vi "运维调试_质控单元.vi"() -> ()   [LabVIEW 2016, in "质控单元.lvlib"]
uses:
  <vilib>/Utility/miscctls.llb/LVPointTypeDef.ctl
  <vilib>/Plasmionique/MB Master/MB_Master_Serial/MB_Master_Serial.lvclass
  C:/Program Files (x86)/National Instruments/LabVIEW 2016/vi.lib/Plasmionique/MB Master/MB_Master/MB_Master.lvclass
  <vilib>/Plasmionique/MB Master/MB Master.lvlib
  <vilib>/ptbypt/NI_PtbyPt.lvlib
panel:
  out "启动模块":T1
  out "COD传感器故障报警":bool
  in  "总氮停止":bool
  in  "总氮排液":bool
  in  "总氮调试":bool
  out "总氮加标回收率":dbl caption="加标回收率" format="%.2f"
  out "总氮加标体积":dbl caption="加标体积" format="%.3f"
  out "总氮母液浓度":dbl caption="加标母液浓度" format="%.3f"
  out "总氮加标水杯定容体积":dbl caption="加标水杯定容体积" format="%.2f"
  out "总氮加标后水样浓度":dbl caption="加标后水样浓度" format="%.3f"
  out "总氮加标前水样浓度":dbl caption="加标前水样浓度" format="%.3f"
  out "总氮检出限":dbl caption="检出限" format="%.3f"
  out "总氮量程":dbl caption="量程" format="%.2f"
  out "总氮状态":u16(ring) caption="状态" items=["待机", "润洗", "进样", "等待取液", "排液"]
  in  "返回":bool
  in  "查看":bool
  out "COD液位传感器":bool
  out "氨氮总磷液位传感器":bool
  out "直接启动":bool
  out "常规启动":bool
  out "总磷总氮传感器故障报警":bool
  out "氨氮传感器故障报警":bool
  out "columns":string[](array[string])
  out "data":T2
  out "氨氮加标回收测完标志":bool
  out "COD加标回收测完标志":bool
  out "氨氮总磷加标回收测完标志":bool
  out "COD平行样测完标志":bool
  out "氨氮总磷平行样测完标志":bool
  out "输出簇 2":T3
  out "常规启动 2":bool
  out "直接启动 2":bool
  out "启动模块 2":cluster{"氨氮1":bool, "总磷1":bool, " COD1":bool}
  in  "停止测量":bool
  out "输出簇":T4
  in  "启动流程":T5(ring)
  in  "加标回收":bool
  in  "平行样测试":bool
  in  "CODMn停止":bool
  in  "CODMn排液":bool
  in  "CODMn调试":bool
  in  "总磷停止":bool
  in  "总磷排液":bool
  in  "总磷调试":bool
  out "COD加标回收率":dbl caption="加标回收率" format="%.2f"
  out "COD加标体积":dbl caption="加标体积" format="%.3f"
  out "COD母液浓度":dbl caption="加标母液浓度" format="%.2f"
  out "COD加标水杯定容体积":dbl caption="加标水杯定容体积" format="%.2f"
  out "COD加标后水样浓度":dbl caption="加标后水样浓度" format="%.2f"
  out "COD加标前水样浓度":dbl caption="加标前水样浓度" format="%.2f"
  out "COD检出限":dbl caption="检出限" format="%.2f"
  out "COD量程":dbl caption="量程" format="%.2f"
  out "COD状态":u16(ring) caption="状态" items=["待机", "润洗", "进样", "等待取液", "排液"]
  out "总磷加标回收率":dbl caption="加标回收率" format="%.2f"
  out "总磷加标体积":dbl caption="加标体积" format="%.3f"
  out "总磷母液浓度":dbl caption="加标母液浓度" format="%.3f"
  out "总磷加标水杯定容体积":dbl caption="加标水杯定容体积" format="%.2f"
  out "总磷加标后水样浓度":dbl caption="加标后水样浓度" format="%.3f"
  out "总磷加标前水样浓度":dbl caption="加标前水样浓度" format="%.3f"
  out "总磷检出限":dbl caption="检出限" format="%.3f"
  out "总磷量程":dbl caption="量程" format="%.2f"
  out "总磷状态":u16(ring) caption="状态" items=["待机", "润洗", "进样", "等待取液", "排液"]
  out "氨氮加标回收率":dbl caption="加标回收率" format="%.2f"
  out "氨氮加标体积":dbl caption="加标体积" format="%.3f"
  out "氨氮母液浓度":dbl caption="加标母液浓度" format="%.3f"
  out "氨氮加标水杯定容体积":dbl caption="加标水杯定容体积" format="%.2f"
  out "氨氮加标后水样浓度":dbl caption="加标后水样浓度" format="%.3f"
  out "氨氮加标前水样浓度":dbl caption="加标前水样浓度" format="%.3f"
  out "氨氮检出限":dbl caption="检出限" format="%.3f"
  out "氨氮量程":dbl caption="量程" format="%.2f"
  out "氨氮状态":u16(ring) caption="状态" items=["待机", "润洗", "进样", "等待取液", "排液"]
  in  "氨氮停止":bool
  in  "氨氮排液":bool
  in  "氨氮调试":bool
  # "总氮质控参数"
  # "%"
  # "mL"
  # "mg/L"
  # "mL"
  # "mg/L"
  # "mg/L"
  # "mg/L"
  # "mg/L"
  # "CODCr质控参数"
  # "%"
  # "mL"
  # "mg/L"
  # "mL"
  # "mg/L"
  # "mg/L"
  # "mg/L"
  # "mg/L"
  # "总磷质控参数"
  # "%"
  # "mL"
  # "mg/L"
  # "mL"
  # "mg/L"
  # "mg/L"
  # "mg/L"
  # "mg/L"
  # "氨氮质控参数"
  # "%"
  # "mL"
  # "mg/L"
  # "mL"
  # "mg/L"
  # "mg/L"
  # "mg/L"
  # "mg/L"
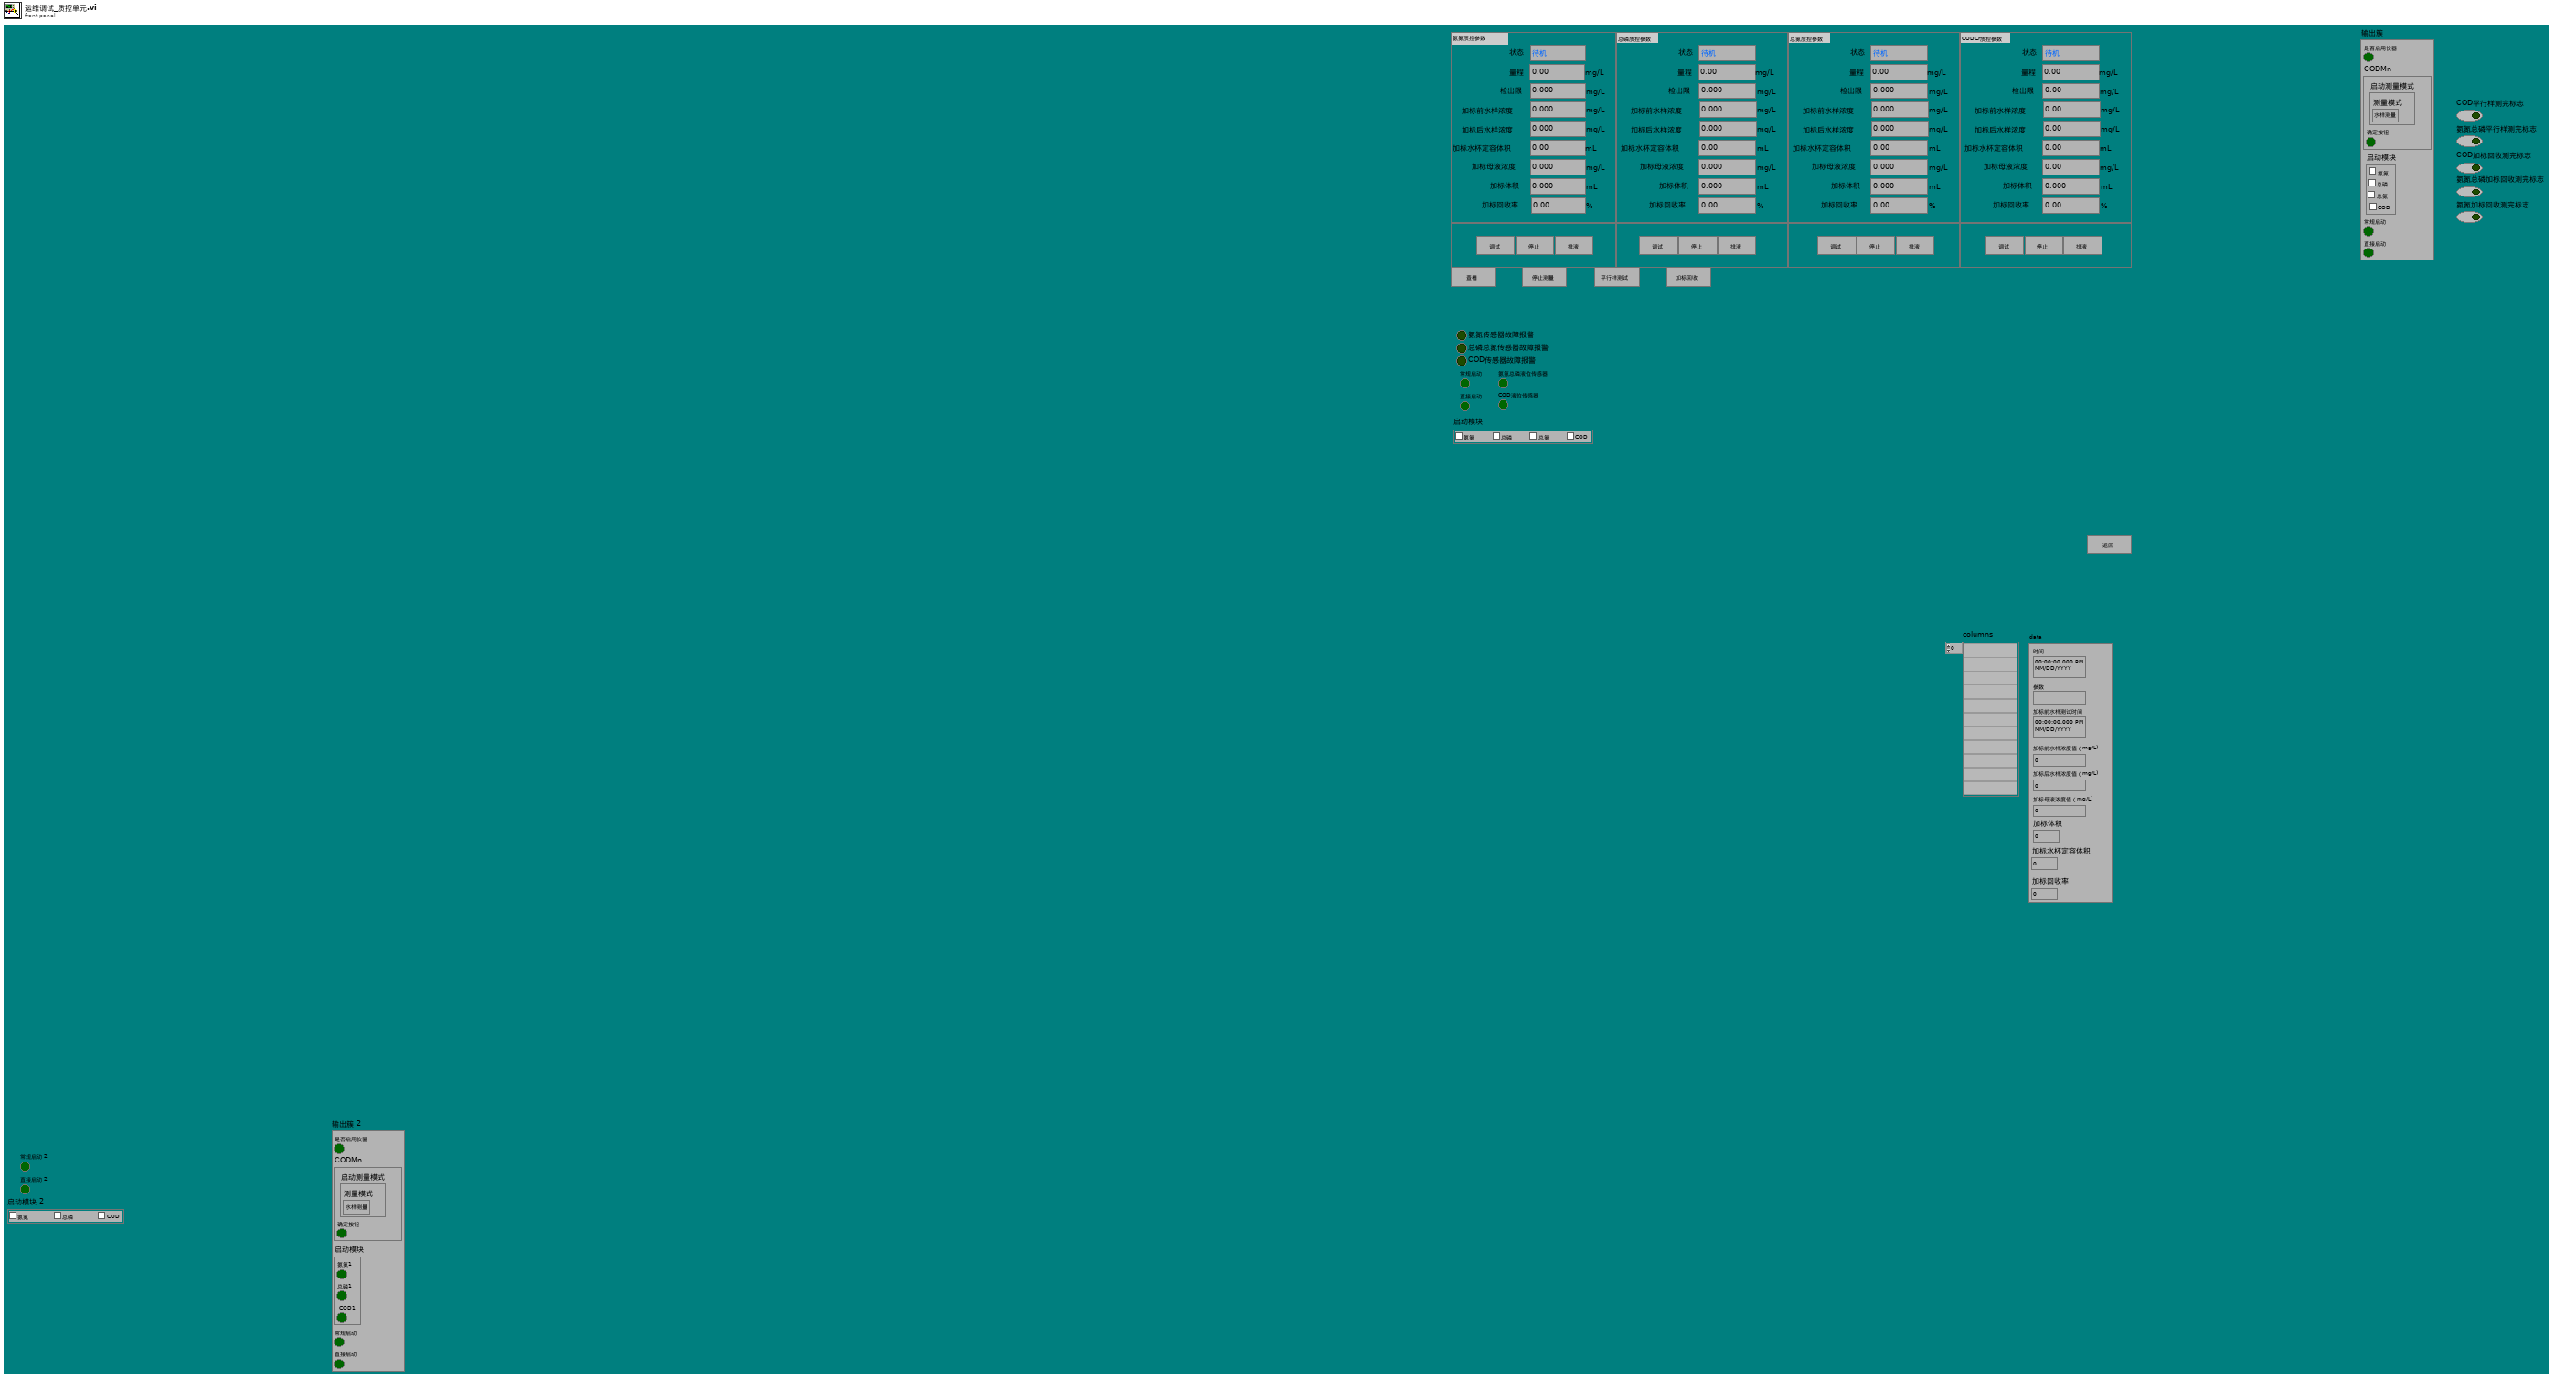
[diagram p1: front panel]
types:
  T1 = cluster{"氨氮":bool, "总磷":bool, "总氮":bool, "COD":bool}
  T2 = cluster{"时间":timestamp, "参数":string, "加标前水样测试时间":timestamp, "加标前水样浓度值（mg/L)":sgl, "加标后水样浓度值（mg/L)":sgl, "加标母液浓度值（mg/L)":sgl, "加标体积":dbl, "加标水杯定容体积":dbl, "加标回收率":dbl}
  T3 = cluster{"是否启用仪器":bool, "CODMn":cluster{"启动测量模式":cluster{"测量模式":enum16{"水样测量", "标样核查", "加标回收", "平行样", "校零", "校标"}}, "确定按钮":bool}, "启动模块":cluster{"氨氮1":bool, "总磷1":bool, " COD1":bool}, "常规启动":bool, "直接启动":bool}
  T4 = cluster{"是否启用仪器":bool, "CODMn":cluster{"启动测量模式":cluster{"测量模式":enum16{"水样测量", "标样核查", "加标回收", "平行样", "校零", "校标"}}, "确定按钮":bool}, "启动模块 3":cluster{"氨氮":bool, "总磷":bool, "总氮":bool, "COD":bool}, "常规启动":bool, "直接启动":bool}
  T5 = enum16{"初始化", "采配水", "测量水样", "加标", "取样测量", "测量结束"}
  T6 = typedef "LVPointTypeDef.ctl" = cluster{"Horizontal":i16, "Vertical":i16}
  T7 = cluster{"baud rate (bps)":u32, "stop bits":u16, "parity":u16, "flow control":u16, "timeout":u32, "retries":i32}
  T8 = cluster{"量程":dbl, "检出限":dbl, "加标前水样浓度":dbl, "加标后水样浓度":dbl, "加标水杯定容体积":dbl, "加标母液浓度":dbl, "加标体积":dbl, "加标回收率":dbl}
  T9 = cluster{"因子编码":u32, "单位":u16, "标样参考值":sgl, "水样数据时间":timestamp, "水样实测值":sgl, "水样数据标识":string, "标样数据时间":timestamp, "标样实测值":sgl, "标样数据标识":string, "空白数据时间":timestamp, "空白实测值":sgl, "空白数据标识":string, "零点核查数据时间":timestamp, "零点核查实测值":sgl, "零点核查数据标识":string, "跨度核查数据时间":timestamp, "跨度核查实测值":sgl, "跨度核查数据标识":string, "加标回收数据时间":timestamp, "加标回收实测值":sgl, "加标回收数据标识":string, "平行样数据时间":timestamp, "平行样实测值":sgl, "平行样数据标识":string, "F0":sgl, "F1":sgl, "F2":sgl, "F3":sgl, "F4":sgl, "F5":sgl, "F6":sgl, "F7":sgl, "温度":sgl, "湿度":sgl, "X值":sgl}
  T10 = cluster{"时间":timestamp, "测量模式":string, "数据类型":string, "检测值":sgl, "单位":string, "数据标识":string, "因子编码":string, "标样参考值":sgl, "ORP-A":sgl, "ORP-B":sgl, "ORP-K":sgl, "COD滴定值":sgl, "高锰酸钾滴定数":sgl, "温度":sgl}
  T11 = enum8{"Enabled", "Disabled", "Disabled and Grayed Out"}
  T12 = cluster{"命令":string, cluster{"starting address":u16, "holding register value":u16}}
  T13 = enum32{"Bad", "Idle", "Run top level", "Running"}
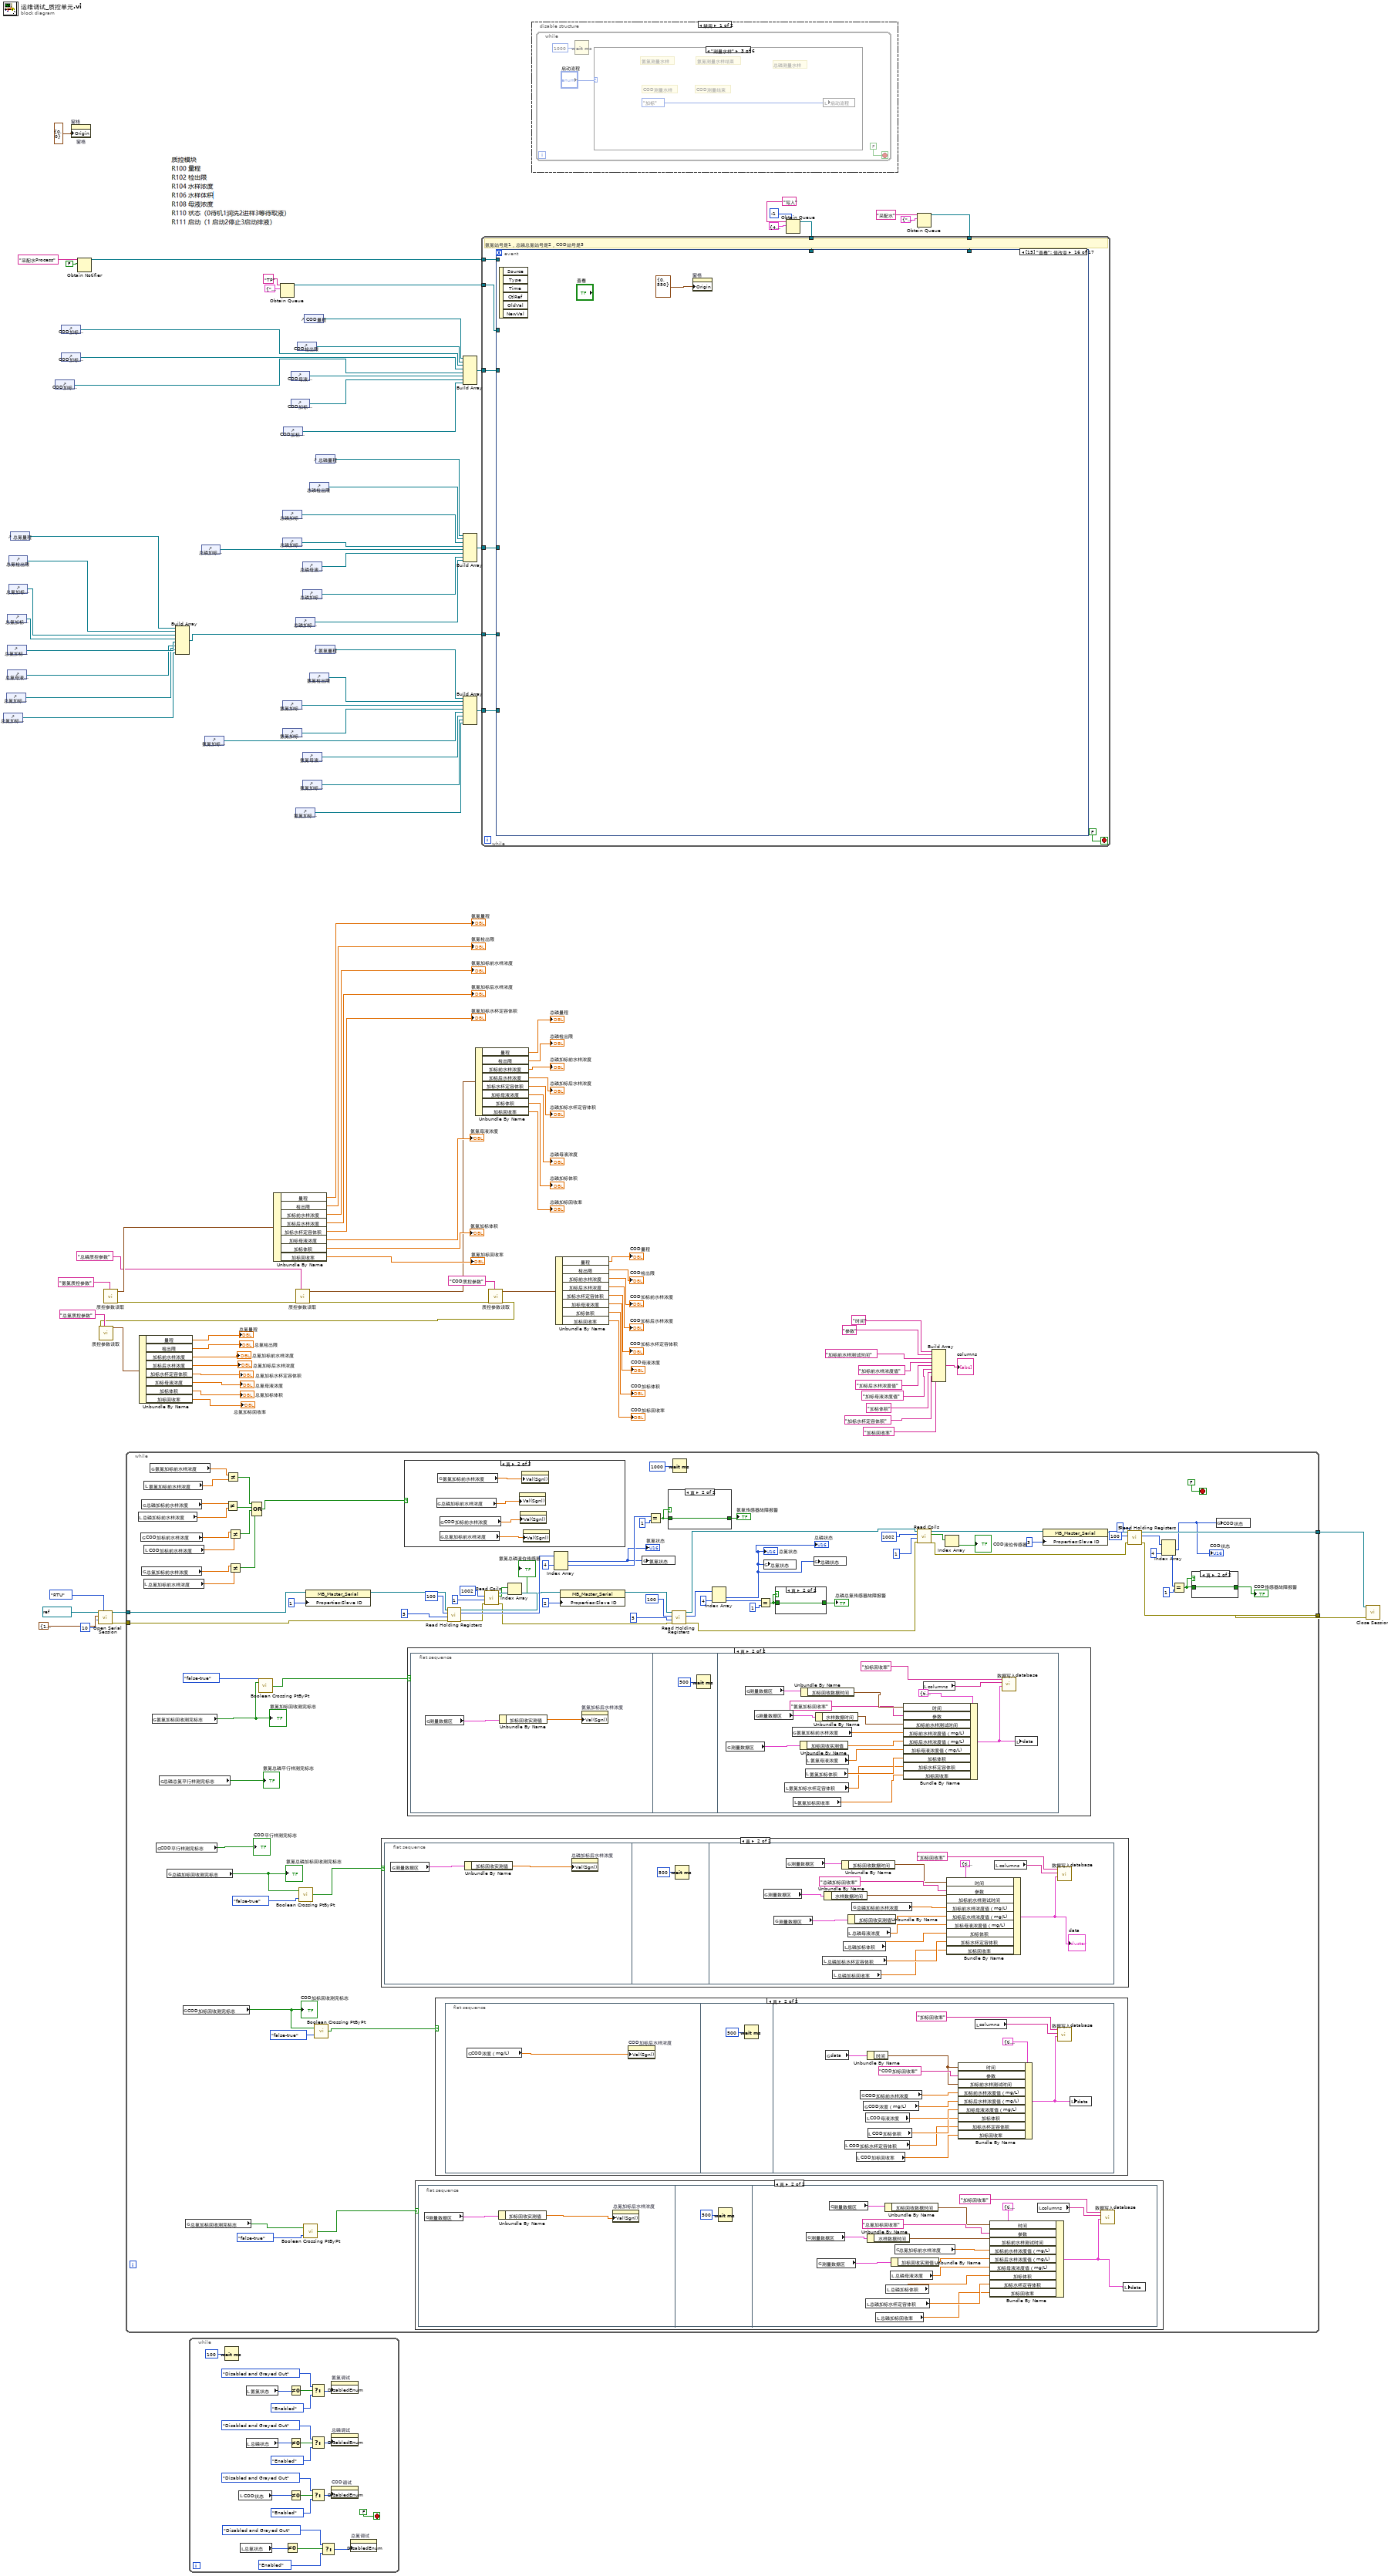
[diagram p0: block diagram]
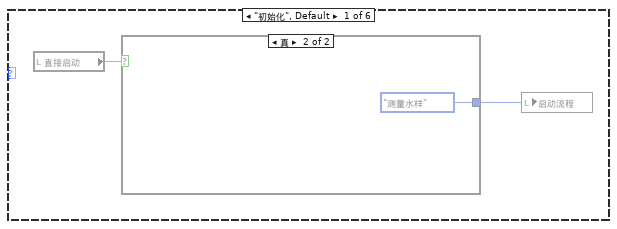
[diagram p2: hidden frame]
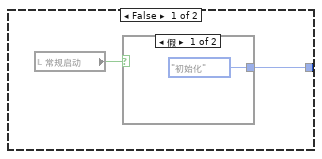
[diagram p3: hidden frame]
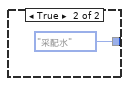
[diagram p4: hidden frame]
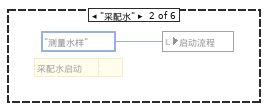
[diagram p5: hidden frame]
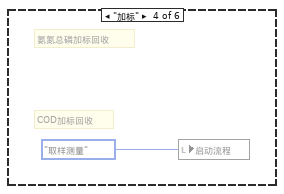
[diagram p6: hidden frame]
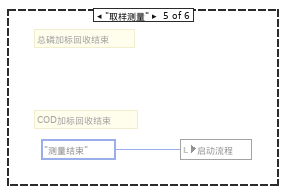
[diagram p7: hidden frame]
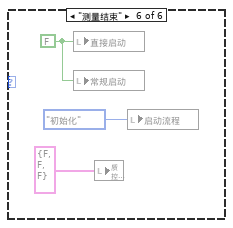
[diagram p8: hidden frame]
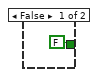
[diagram p11: hidden frame]
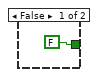
[diagram p16: hidden frame]
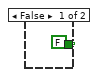
[diagram p17: hidden frame]
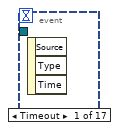
[diagram p18: hidden frame]
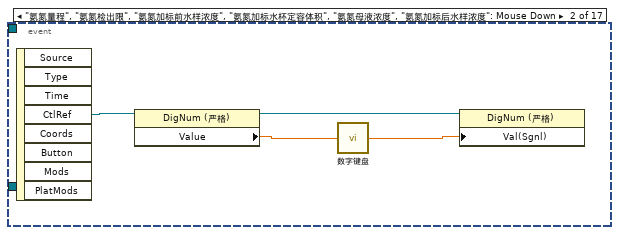
[diagram p19: hidden frame]
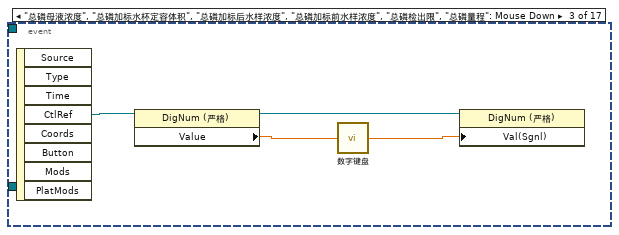
[diagram p20: hidden frame]
diagram:
  n1 = control-ref of="总氮加标回收率"() -> (w17:refnum<vi>)
  n2 = control-ref of="总氮加标体积"() -> (w18:refnum<vi>)
  n3 = control-ref of="总氮加标水杯定容体积"() -> (w20:refnum<vi>)
  n4 = control-ref of="总氮加标后水样浓度"() -> (w21:refnum<vi>)
  n5 = control-ref of="总氮母液浓度"() -> (w19:refnum<vi>)
  n6 = control-ref of="总氮检出限"() -> (w23:refnum<vi>)
  n7 = control-ref of="总氮加标前水样浓度"() -> (w22:refnum<vi>)
  n8 = control-ref of="总氮量程"() -> (w24:refnum<vi>)
  n9 = control-ref of="COD加标水杯定容体积"() -> (w57:refnum<vi>)
  n10 = control-ref of="COD加标前水样浓度"() -> (w59:refnum<vi>)
  n11 = control-ref of="COD加标后水样浓度"() -> (w58:refnum<vi>)
  n12 = property on="窗格" class="Pane"("Origin"=T6 {"Horizontal"=0, "Vertical"=0} ("原点")) -> ()  [unwired: 2 in, 2 out]
  n13 = property on="窗格" class="Pane"("Origin"=T6 {"Horizontal"=0, "Vertical"=0} ("原点")) -> ()  [unwired: 2 in, 2 out]
  n14 = Obtain Notifier(name (unnamed)="采配水Process" ("名称（未命名）"), notification data type=FALSE) -> (notifier out=w43:refnum<notifier>)  [unwired: 2 in, 2 out]
  n15 = call <vilib>:"Open Serial Session.vi"("Mode (RTU)"=enum16{"RTU", "ASCII"}."RTU", "Slave ID"=u8 10, "Serial Config"=T7 {"baud rate (bps)"=115200, "stop bits"=10, "parity"=0, "flow control"=0, "timeout"=100, "retries"=1}, "VISA Resource"=refnum<visa-resource-name> "COM6") -> ("Error out"=w51:errorcluster, "MB_Serial session"=w52:refnum<class "MB_Master_Serial.lvclass">)  [unwired: 6 in]
  n16 = call "质控参数读取.vi"("section"="氨氮质控参数") -> ("error out"=w82:errorcluster, "参数"=w101:T8)  [unwired: 9 in]
  n17 = while {
    tunnel: w52 -> [w192]
    tunnel: w51 -> [w191]
    tunnel: [w125] -> w50
    tunnel: [w124] -> w1
    stop <- FALSE stop-if-true
    n18 = local read "总磷加标前水样浓度"() -> (w166:dbl)
    n19 = global read "水样浓度全局.vi" "COD加标前水样浓度"() -> (w165:dbl)
    n20 = global read "水样浓度全局.vi" "总磷加标前水样浓度"() -> (w167:dbl)
    n21 = global read "水样浓度全局.vi" "总氮加标前水样浓度"() -> (w136:dbl)
    n22 = local read "总氮加标前水样浓度"() -> (w137:dbl)
    n23 = local read "氨氮加标前水样浓度"() -> (w168:dbl)
    n24 = local read "COD加标前水样浓度"() -> (w164:dbl)
    n25 = global read "水样浓度全局.vi" "氨氮加标前水样浓度"() -> (w169:dbl)
    n26 = global read "质控测完标志全局 1.vi" "氨氮加标回收测完标志"() -> (w157:bool)
    "氨氮加标回收测完标志" <- w157
    n27 = global read "质控测完标志全局 1.vi" "COD平行样测完标志"() -> (→"COD平行样测完标志":bool)
    n28 = global read "质控测完标志全局 1.vi" "总磷总氮平行样测完标志"() -> (→"氨氮总磷平行样测完标志":bool)
    n29 = global read "质控测完标志全局 1.vi" "总磷加标回收测完标志"() -> (w116:bool)
    "氨氮总磷加标回收测完标志" <- w116
    n30 = global read "质控测完标志全局 1.vi" "COD加标回收测完标志"() -> (w152:bool)
    "COD加标回收测完标志" <- w152
    n31 = global read "质控测完标志全局 1.vi" "总氮加标回收测完标志"() -> (w114:bool)
    n32 = Not Equal?(x=w167, y=w166) -> (x != y?=w161:bool)
    n33 = Not Equal?(x=w169, y=w168) -> (x != y?=w163:bool)
    n34 = Not Equal?(x=w165, y=w164) -> (x != y?=w160:bool)
    n35 = Not Equal?(x=w136, y=w137) -> (x != y?=w135:bool)
    n36 = Compound Arithmetic op=OR ("复合运算")(w163, w161, w160, w135) -> (w162:bool)
    n37 = call <vilib>:"Boolean Crossing PtByPt.vi"("direction"=enum16{"either", "false-true", "true-false"}."false-true", "input"=w157) -> ("crossing"=w156:bool)  [unwired: 1 in]
    n38 = call <vilib>:"Boolean Crossing PtByPt.vi"("direction"=enum16{"either", "false-true", "true-false"}."false-true", "input"=w116) -> ("crossing"=w153:bool)  [unwired: 1 in]
    n39 = call <vilib>:"Boolean Crossing PtByPt.vi"("direction"=enum16{"either", "false-true", "true-false"}."false-true", "input"=w114) -> ("crossing"=w113:bool)  [unwired: 1 in]
    n40 = property class="MB_Master_Serial"(reference=w192, "Properties:Slave ID"=u8 1 ("Slave ID")) -> (reference out=w181:refnum<class "MB_Master_Serial.lvclass">)  [unwired: 1 in, 1 out]
    n41 = call <vilib>:"Boolean Crossing PtByPt.vi"("direction"=enum16{"either", "false-true", "true-false"}."false-true", "input"=w152) -> ("crossing"=w150:bool)  [unwired: 1 in]
    n42 = case shown="真" w153 {
      frame False {
      }
      frame True {
        n43 = flat-sequence {
          frame #0 {
            n44 = global read "VAR总磷氨氮全局变量.vi" "测量数据区"() -> (w232:T9)
            n45 = Unbundle By Name(w232) -> ("加标回收实测值"=w231:sgl)
            n46 = property on="总磷加标后水样浓度" class="DigNum (严格)"("Val(Sgnl)"=w231) -> ()  [unwired: 2 in, 2 out]
          }
          frame #1 {
            n47 = Wait (ms)(milliseconds to wait=u32 500 ("等待时间（毫秒）")) -> ()  [unwired: 1 out]
          }
          frame #2 {
            n48 = global read "VAR总磷氨氮全局变量.vi" "测量数据区"() -> (w235:T9)
            n49 = global read "VAR总磷氨氮全局变量.vi" "测量数据区"() -> (w246:T9)
            n50 = global read "VAR总磷氨氮全局变量.vi" "测量数据区"() -> (w239:T9)
            n51 = local read "总磷加标水杯定容体积"() -> (w242:dbl)
            n52 = Unbundle By Name(w235) -> ("水样数据时间"=w234:timestamp)
            n53 = local read "总磷加标回收率"() -> (w241:dbl)
            n54 = Unbundle By Name(w239) -> ("加标回收数据时间"=w236:timestamp)
            n55 = local read "总磷加标体积"() -> (w243:dbl)
            n56 = local read "总磷母液浓度"() -> (w244:dbl)
            n57 = Unbundle By Name(w246) -> ("加标回收实测值"=w245:sgl)
            n58 = global read "水样浓度全局.vi" "总磷加标前水样浓度"() -> (w247:dbl)
            n59 = Bundle By Name(cluster=T2 {"时间"=timestamp(0 s since 1904-01-01), "参数"="", "加标前水样测试时间"=timestamp(0 s since 1904-01-01), "加标前水样浓度值（mg/L)"=0.0, "加标后水样浓度值（mg/L)"=0.0, "加标母液浓度值（mg/L)"=0.0, "加标体积"=0.0, "加标水杯定容体积"=0.0, "加标回收率"=0.0} ("data"), "时间"=w236, "参数"="总磷加标回收率" ("table"), "加标前水样测试时间"=w234, "加标前水样浓度值（mg/L)"=w247, "加标后水样浓度值（mg/L)"=w245, "加标母液浓度值（mg/L)"=w244, "加标体积"=w243, "加标水杯定容体积"=w242, "加标回收率"=w241) -> (w240:T2)
            "data" <- w240
            n60 = local read "columns"() -> (w248:string[])
            n61 = call "数据写入database.vi"("data"=w240, "columns"=w248, "table"="加标回收率") -> ()  [unwired: 9 in]
          }
        }
      }
    }
    n62 = case shown="真" w162 {
      frame False {
      }
      frame True {
        n63 = global read "水样浓度全局.vi" "总磷加标前水样浓度"() -> (w271:dbl)
        n64 = global read "水样浓度全局.vi" "氨氮加标前水样浓度"() -> (w272:dbl)
        n65 = global read "水样浓度全局.vi" "COD加标前水样浓度"() -> (w270:dbl)
        n66 = global read "水样浓度全局.vi" "总氮加标前水样浓度"() -> (w269:dbl)
        n67 = property on="总磷加标前水样浓度" class="DigNum (严格)"("Val(Sgnl)"=w271) -> ()  [unwired: 2 in, 2 out]
        n68 = property on="COD加标前水样浓度" class="DigNum (严格)"("Val(Sgnl)"=w270) -> ()  [unwired: 2 in, 2 out]
        n69 = property on="氨氮加标前水样浓度" class="DigNum (严格)"("Val(Sgnl)"=w272) -> ()  [unwired: 2 in, 2 out]
        n70 = property on="总氮加标前水样浓度" class="DigNum (严格)"("Val(Sgnl)"=w269) -> ()  [unwired: 2 in, 2 out]
      }
    }
    n71 = case shown="真" w156 {
      frame False {
      }
      frame True {
        n72 = flat-sequence {
          frame #0 {
            n73 = global read "VAR总磷氨氮全局变量.vi" "测量数据区"() -> (w251:T9)
            n74 = Unbundle By Name(w251) -> ("加标回收实测值"=w250:sgl)
            n75 = property on="氨氮加标后水样浓度" class="DigNum (严格)"("Val(Sgnl)"=w250) -> ()  [unwired: 2 in, 2 out]
          }
          frame #1 {
            n76 = Wait (ms)(milliseconds to wait=u32 500 ("等待时间（毫秒）")) -> ()  [unwired: 1 out]
          }
          frame #2 {
            n77 = global read "VAR总磷氨氮全局变量.vi" "测量数据区"() -> (w264:T9)
            n78 = global read "VAR总磷氨氮全局变量.vi" "测量数据区"() -> (w266:T9)
            n79 = global read "VAR总磷氨氮全局变量.vi" "测量数据区"() -> (w258:T9)
            n80 = local read "氨氮加标水杯定容体积"() -> (w260:dbl)
            n81 = global read "水样浓度全局.vi" "氨氮加标前水样浓度"() -> (w265:dbl)
            n82 = local read "氨氮加标回收率"() -> (w259:dbl)
            n83 = Unbundle By Name(w264) -> ("加标回收实测值"=w263:sgl)
            n84 = Unbundle By Name(w266) -> ("加标回收数据时间"=w256:timestamp)
            n85 = local read "氨氮加标体积"() -> (w261:dbl)
            n86 = local read "氨氮母液浓度"() -> (w262:dbl)
            n87 = Unbundle By Name(w258) -> ("水样数据时间"=w254:timestamp)
            n88 = Bundle By Name(cluster=T2 {"时间"=timestamp(0 s since 1904-01-01), "参数"="", "加标前水样测试时间"=timestamp(0 s since 1904-01-01), "加标前水样浓度值（mg/L)"=0.0, "加标后水样浓度值（mg/L)"=0.0, "加标母液浓度值（mg/L)"=0.0, "加标体积"=0.0, "加标水杯定容体积"=0.0, "加标回收率"=0.0} ("data"), "时间"=w256, "参数"="氨氮加标回收率" ("table"), "加标前水样测试时间"=w254, "加标前水样浓度值（mg/L)"=w265, "加标后水样浓度值（mg/L)"=w263, "加标母液浓度值（mg/L)"=w262, "加标体积"=w261, "加标水杯定容体积"=w260, "加标回收率"=w259) -> (w253:T2)
            n89 = local read "columns"() -> (w267:string[])
            n90 = call "数据写入database.vi"("data"=w253, "columns"=w267, "table"="加标回收率") -> ()  [unwired: 9 in]
            n91 = local write "data"(w253) -> ()
          }
        }
      }
    }
    n92 = case shown="真" w113 {
      frame False {
      }
      frame True {
        n93 = flat-sequence {
          frame #0 {
            n94 = global read "VAR总磷氨氮全局变量.vi" "测量数据区"() -> (w196:T9)
            n95 = Unbundle By Name(w196) -> ("加标回收实测值"=w195:sgl)
            n96 = property on="总氮加标后水样浓度" class="DigNum (严格)"("Val(Sgnl)"=w195) -> ()  [unwired: 2 in, 2 out]
          }
          frame #1 {
            n97 = Wait (ms)(milliseconds to wait=u32 500 ("等待时间（毫秒）")) -> ()  [unwired: 1 out]
          }
          frame #2 {
            n98 = global read "VAR总磷氨氮全局变量.vi" "测量数据区"() -> (w200:T9)
            n99 = global read "VAR总磷氨氮全局变量.vi" "测量数据区"() -> (w210:T9)
            n100 = global read "VAR总磷氨氮全局变量.vi" "测量数据区"() -> (w204:T9)
            n101 = local read "总磷加标水杯定容体积"() -> (w206:dbl)
            n102 = Unbundle By Name(w200) -> ("水样数据时间"=w199:timestamp)
            n103 = local read "总磷加标回收率"() -> (w205:dbl)
            n104 = Unbundle By Name(w204) -> ("加标回收数据时间"=w201:timestamp)
            n105 = local read "总磷加标体积"() -> (w207:dbl)
            n106 = local read "总磷母液浓度"() -> (w208:dbl)
            n107 = Unbundle By Name(w210) -> ("加标回收实测值"=w209:sgl)
            n108 = global read "水样浓度全局.vi" "总氮加标前水样浓度"() -> (w211:dbl)
            n109 = Bundle By Name(cluster=T2 {"时间"=timestamp(0 s since 1904-01-01), "参数"="", "加标前水样测试时间"=timestamp(0 s since 1904-01-01), "加标前水样浓度值（mg/L)"=0.0, "加标后水样浓度值（mg/L)"=0.0, "加标母液浓度值（mg/L)"=0.0, "加标体积"=0.0, "加标水杯定容体积"=0.0, "加标回收率"=0.0} ("data"), "时间"=w201, "参数"="总氮加标回收率" ("table"), "加标前水样测试时间"=w199, "加标前水样浓度值（mg/L)"=w211, "加标后水样浓度值（mg/L)"=w209, "加标母液浓度值（mg/L)"=w208, "加标体积"=w207, "加标水杯定容体积"=w206, "加标回收率"=w205) -> (w198:T2)
            n110 = local read "columns"() -> (w212:string[])
            n111 = call "数据写入database.vi"("data"=w198, "columns"=w212, "table"="加标回收率") -> ()  [unwired: 9 in]
            n112 = local write "data"(w198) -> ()
          }
        }
      }
    }
    n113 = case shown="真" w150 {
      frame False {
      }
      frame True {
        n114 = flat-sequence {
          frame #0 {
            n115 = global read "COD浓度全局变量.vi" "COD浓度（mg/L)"() -> (w216:dbl)
            n116 = property on="COD加标后水样浓度" class="DigNum (严格)"("Val(Sgnl)"=w216) -> ()  [unwired: 2 in, 2 out]
          }
          frame #1 {
            n117 = Wait (ms)(milliseconds to wait=u32 500 ("等待时间（毫秒）")) -> ()  [unwired: 1 out]
          }
          frame #2 {
            n118 = global read "COD读取DATA全局.vi" "data"() -> (w228:T10)
            n119 = local read "COD加标水杯定容体积"() -> (w223:dbl)
            n120 = local read "COD加标回收率"() -> (w222:dbl)
            n121 = global read "水样浓度全局.vi" "COD加标前水样浓度"() -> (w227:dbl)
            n122 = global read "COD浓度全局变量.vi" "COD浓度（mg/L)"() -> (w226:dbl)
            n123 = local read "COD母液浓度"() -> (w225:dbl)
            n124 = Unbundle By Name(w228) -> ("时间"=w218:timestamp)
            n125 = local read "COD加标体积"() -> (w224:dbl)
            n126 = Bundle By Name(cluster=T2 {"时间"=timestamp(0 s since 1904-01-01), "参数"="", "加标前水样测试时间"=timestamp(0 s since 1904-01-01), "加标前水样浓度值（mg/L)"=0.0, "加标后水样浓度值（mg/L)"=0.0, "加标母液浓度值（mg/L)"=0.0, "加标体积"=0.0, "加标水杯定容体积"=0.0, "加标回收率"=0.0} ("data"), "时间"=w218, "参数"="COD加标回收率" ("table"), "加标前水样测试时间"=w218, "加标前水样浓度值（mg/L)"=w227, "加标后水样浓度值（mg/L)"=w226, "加标母液浓度值（mg/L)"=w225, "加标体积"=w224, "加标水杯定容体积"=w223, "加标回收率"=w222) -> (w221:T2)
            n127 = local read "columns"() -> (w229:string[])
            n128 = call "数据写入database.vi"("data"=w221, "columns"=w229, "table"="加标回收率") -> ()  [unwired: 9 in]
            n129 = local write "data"(w221) -> ()
          }
        }
      }
    }
    n130 = call <vilib>:"Read Holding Registers.vi"("error in (no error)"=w191, "quantity"=u16 5, "starting address"=u16 100, "MB session in"=w181) -> ("error out"=w145:errorcluster, "Registers"=w188:u16[], "MB session out"=w184:refnum<class "MB_Master_Serial.lvclass">)  [unwired: 5 in]
    n131 = call <vilib>:"Read Coils.vi"("error in (no error)"=w145, "quantity"=u16 1, "starting address"=u16 1002, "MB session in"=w184) -> ("error out"=w144:errorcluster, "Coils"=w146:bool[], "MB session out"=w149:refnum<class "MB_Master_Serial.lvclass">)  [unwired: 5 in]
    n132 = Index Array(array=w146) -> (element=→"氨氮总磷液位传感器":bool)  [unwired: 1 in]
    n133 = Index Array(array=w188, index #2=4 ("索引")) -> (element #1=w134:u16, element #2=w178:u16)  [unwired: 2 in, 1 out]
    "氨氮状态" <- w134
    n134 = property class="MB_Master_Serial"(reference=w149, "Properties:Slave ID"=u8 2 ("Slave ID")) -> (reference out=w183:refnum<class "MB_Master_Serial.lvclass">)  [unwired: 1 in, 1 out]
    n135 = global write "氨氮加标回收状态全局变量.vi" "氨氮状态"(w134) -> ()
    n136 = Equal?(x=w178, y=u16 1) -> (x = y?=w175:bool)
    n137 = case shown="真" w175 {
      tunnel: w175 -> [_ w276]
      tunnel: [FALSE w276] -> w176
      frame False {
      }
      frame True {
      }
    }
    "氨氮传感器故障报警" <- w176
    n138 = call <vilib>:"Read Holding Registers.vi"("error in (no error)"=w144, "quantity"=u16 5, "starting address"=u16 100, "MB session in"=w183) -> ("error out"=w138:errorcluster, "Registers"=w187:u16[], "MB session out"=w132:refnum<class "MB_Master_Serial.lvclass">)  [unwired: 5 in]
    n139 = Wait (ms)(milliseconds to wait=u32 1000 ("等待时间（毫秒）")) -> ()  [unwired: 1 out]
    n140 = Index Array(array=w187, index #2=4 ("索引")) -> (element #1=w133:u16, element #2=w172:u16)  [unwired: 1 in]
    "总磷状态" <- w133
    "总氮状态" <- w133
    n141 = Equal?(x=w172, y=u16 1) -> (x = y?=w170:bool)
    n142 = global write "氨氮加标回收状态全局变量.vi" "总氮状态"(w133) -> ()
    n143 = case shown="真" w170 {
      tunnel: w170 -> [_ w274]
      tunnel: [FALSE w274] -> w171
      frame False {
      }
      frame True {
      }
    }
    "总磷总氮传感器故障报警" <- w171
    n144 = global write "氨氮加标回收状态全局变量.vi" "总磷状态"(w133) -> ()
    n145 = call <vilib>:"Read Coils.vi"("error in (no error)"=w138, "quantity"=u16 1, "starting address"=u16 1002, "MB session in"=w132) -> ("error out"=w126:errorcluster, "Coils"=w140:bool[], "MB session out"=w131:refnum<class "MB_Master_Serial.lvclass">)  [unwired: 5 in]
    n146 = Index Array(array=w140) -> (element=→"COD液位传感器":bool)  [unwired: 1 in]
    n147 = property class="MB_Master_Serial"(reference=w131, "Properties:Slave ID"=u8 3 ("Slave ID")) -> (reference out=w129:refnum<class "MB_Master_Serial.lvclass">)  [unwired: 1 in, 1 out]
    n148 = call <vilib>:"Read Holding Registers.vi"("error in (no error)"=w126, "quantity"=u16 5, "starting address"=u16 100, "MB session in"=w129) -> ("error out"=w125:errorcluster, "Registers"=w123:u16[], "MB session out"=w124:refnum<class "MB_Master_Serial.lvclass">)  [unwired: 5 in]
    n149 = Index Array(array=w123, index #2=4 ("索引")) -> (element #1=w121:u16, element #2=w118:u16)  [unwired: 1 in]
    "COD状态" <- w121
    n150 = Equal?(x=w118, y=u16 1) -> (x = y?=w120:bool)
    n151 = case shown="真" w120 {
      tunnel: w120 -> [_ w215]
      tunnel: [FALSE w215] -> w117
      frame False {
      }
      frame True {
      }
    }
    "COD传感器故障报警" <- w117
    n152 = global write "氨氮加标回收状态全局变量.vi" "COD状态"(w121) -> ()
  }
  n153 = Build Array(w24, w23, w22, w21, w20, w19, w18, w17) -> (w16:refnum<vi>[])
  n154 = while {
    stop <- FALSE stop-if-true
    n155 = Wait (ms)(milliseconds to wait=u32 100 ("等待时间（毫秒）")) -> ()  [unwired: 1 out]
    n156 = local read "COD状态"() -> (w283:u16)
    n157 = local read "总氮状态"() -> (w281:u16)
    n158 = local read "氨氮状态"() -> (w297:u16)
    n159 = local read "总磷状态"() -> (w288:u16)
    n160 = Not Equal To 0?(x=w281) -> (x != 0?=w280:bool)
    n161 = Not Equal To 0?(x=w297) -> (x != 0?=w296:bool)
    n162 = Not Equal To 0?(x=w288) -> (x != 0?=w290:bool)
    n163 = Not Equal To 0?(x=w283) -> (x != 0?=w287:bool)
    n164 = Select(t=T11."Disabled and Grayed Out" ("禁用"), s=w296, f=T11."Enabled") -> (s? t:f=w293:T11)
    n165 = Select(t=T11."Disabled and Grayed Out" ("禁用"), s=w290, f=T11."Enabled") -> (s? t:f=w289:T11)
    n166 = Select(t=T11."Disabled and Grayed Out" ("禁用"), s=w287, f=T11."Enabled") -> (s? t:f=w284:T11)
    n167 = Select(t=T11."Disabled and Grayed Out" ("禁用"), s=w280, f=T11."Enabled") -> (s? t:f=w277:T11)
    n168 = property on="氨氮调试" class="Bool"("DisabledEnum"=w293) -> ()  [unwired: 2 in, 2 out]
    n169 = property on="总磷调试" class="Bool"("DisabledEnum"=w289) -> ()  [unwired: 2 in, 2 out]
    n170 = property on="COD调试" class="Bool"("DisabledEnum"=w284) -> ()  [unwired: 2 in, 2 out]
    n171 = property on="总氮调试" class="Bool"("DisabledEnum"=w277) -> ()  [unwired: 2 in, 2 out]
  }
  n172 = control-ref of="总磷加标水杯定容体积"() -> (w66:refnum<vi>)
  n173 = control-ref of="氨氮加标水杯定容体积"() -> (w108:refnum<vi>)
  n174 = Unbundle By Name(w101) -> ("量程"=→"氨氮量程":dbl, "检出限"=→"氨氮检出限":dbl, "加标前水样浓度"=→"氨氮加标前水样浓度":dbl, "加标后水样浓度"=→"氨氮加标后水样浓度":dbl, "加标水杯定容体积"=→"氨氮加标水杯定容体积":dbl, "加标母液浓度"=→"氨氮母液浓度":dbl, "加标体积"=→"氨氮加标体积":dbl, "加标回收率"=→"氨氮加标回收率":dbl)
  n175 = Obtain Queue(name (unnamed)="TP" ("名称（未命名）"), element data type=cluster{"命令":string, "data":variant} {"命令"="", "data"=variant}) -> (queue out=w33:refnum<queue>)  [unwired: 3 in, 2 out]
  n176 = control-ref of="总磷加标前水样浓度"() -> (w68:refnum<vi>)
  n177 = control-ref of="总磷加标后水样浓度"() -> (w67:refnum<vi>)
  n178 = control-ref of="氨氮加标前水样浓度"() -> (w109:refnum<vi>)
  n179 = control-ref of="氨氮加标后水样浓度"() -> (w105:refnum<vi>)
  n180 = control-ref of="COD加标回收率"() -> (w54:refnum<vi>)
  n181 = control-ref of="COD母液浓度"() -> (w56:refnum<vi>)
  n182 = control-ref of="COD加标体积"() -> (w55:refnum<vi>)
  n183 = call "质控参数读取.vi"("section"="总磷质控参数", "error in (no error)"=w82) -> ("error out"=w79:errorcluster, "参数"=w91:T8)  [unwired: 8 in]
  n184 = control-ref of="总磷加标回收率"() -> (w64:refnum<vi>)
  n185 = control-ref of="氨氮加标回收率"() -> (w103:refnum<vi>)
  n186 = control-ref of="COD检出限"() -> (w60:refnum<vi>)
  n187 = control-ref of="总磷母液浓度"() -> (w65:refnum<vi>)
  n188 = control-ref of="总磷加标体积"() -> (w63:refnum<vi>)
  n189 = control-ref of="氨氮母液浓度"() -> (w107:refnum<vi>)
  n190 = control-ref of="氨氮加标体积"() -> (w104:refnum<vi>)
  n191 = control-ref of="COD量程"() -> (w61:refnum<vi>)
  n192 = control-ref of="总磷检出限"() -> (w69:refnum<vi>)
  n193 = control-ref of="氨氮检出限"() -> (w110:refnum<vi>)
  n194 = control-ref of="总磷量程"() -> (w70:refnum<vi>)
  n195 = control-ref of="氨氮量程"() -> (w111:refnum<vi>)
  n196 = Build Array(w61, w60, w59, w58, w57, w56, w55, w54) -> (w53:refnum<vi>[])
  n197 = Build Array(w70, w69, w68, w67, w66, w65, w63, w64) -> (w62:refnum<vi>[])
  n198 = Build Array(w111, w110, w109, w105, w108, w107, w104, w103) -> (w106:refnum<vi>[])
  n199 = Unbundle By Name(w91) -> ("量程"=→"总磷量程":dbl, "检出限"=→"总磷检出限":dbl, "加标前水样浓度"=→"总磷加标前水样浓度":dbl, "加标后水样浓度"=→"总磷加标后水样浓度":dbl, "加标水杯定容体积"=→"总磷加标水杯定容体积":dbl, "加标母液浓度"=→"总磷母液浓度":dbl, "加标体积"=→"总磷加标体积":dbl, "加标回收率"=→"总磷加标回收率":dbl)
  n200 = call "质控参数读取.vi"("section"="COD质控参数", "error in (no error)"=w79) -> ("error out"=w14:errorcluster, "参数"=w81:T8)  [unwired: 8 in]
  n201 = call "质控参数读取.vi"("section"="总氮质控参数", "error in (no error)"=w14) -> ("参数"=w13:T8)  [unwired: 8 in, 1 out]
  n202 = Unbundle By Name(w13) -> ("量程"=→"总氮量程":dbl, "检出限"=→"总氮检出限":dbl, "加标前水样浓度"=→"总氮加标前水样浓度":dbl, "加标后水样浓度"=→"总氮加标后水样浓度":dbl, "加标水杯定容体积"=→"总氮加标水杯定容体积":dbl, "加标母液浓度"=→"总氮母液浓度":dbl, "加标体积"=→"总氮加标体积":dbl, "加标回收率"=→"总氮加标回收率":dbl)
  n203 = disable-structure shown="禁用" {
    frame Disabled {
      n204 = while {
        stop <- FALSE stop-if-true
        n205 = Wait (ms)(milliseconds to wait=u32 1000 ("等待时间（毫秒）")) -> ()  [unwired: 1 out]
        n206 = case shown="\"测量水样\"" "启动流程" {
          frame "初始化", Default {
            n207 = local read "直接启动"() -> (w303:bool)
            n208 = case shown="真" w303 {
              tunnel: [w304 T5."测量水样" ("启动流程")] -> w302
              frame False {
                n209 = local read "常规启动"() -> (w305:bool)
                n210 = case shown="假" w305 {
                  tunnel: [T5."初始化" ("启动流程") T5."采配水" ("启动流程")] -> w304
                  frame False {
                  }
                  frame True {
                  }
                }
              }
              frame True {
              }
            }
            n211 = local write "启动流程"(w302) -> ()
          }
          frame "采配水" {
            # "采配水启动结束"
            # "采配水启动"
            n212 = local write "启动流程"(T5."测量水样" ("启动流程")) -> ()
          }
          frame "测量水样" {
            # "总磷测量水样"
            # "COD测量结束"
            # "总磷测量结束"
            # "氨氮测量水样结束"
            # "COD测量水样"
            # "氨氮测量水样"
            n213 = local write "启动流程"(T5."加标" ("启动流程")) -> ()
          }
          frame "加标" {
            # "COD加标回收"
            # "氨氮总磷加标回收"
            n214 = local write "启动流程"(T5."取样测量" ("启动流程")) -> ()
          }
          frame "取样测量" {
            # "COD加标回收结束"
            # "总磷加标回收结束"
            n215 = local write "启动流程"(T5."测量结束" ("启动流程")) -> ()
          }
          frame "测量结束" {
            w314 = FALSE ("直接启动")
            n216 = local write "直接启动"(w314) -> ()
            n217 = local write "常规启动"(w314) -> ()
            n218 = local write item#-1(cluster{"氨氮1":bool, "总磷1":bool, " COD1":bool} {"氨氮1"=FALSE, "总磷1"=FALSE, " COD1"=FALSE} ("启动模块")) -> ()
            n219 = local write "启动流程"(T5."初始化" ("启动流程")) -> ()
          }
        }
      }
    }
    frame Enabled {
    }
  }
  n220 = Unbundle By Name(w81) -> ("量程"=→"COD量程":dbl, "检出限"=→"COD检出限":dbl, "加标前水样浓度"=→"COD加标前水样浓度":dbl, "加标后水样浓度"=→"COD加标后水样浓度":dbl, "加标水杯定容体积"=→"COD加标水杯定容体积":dbl, "加标母液浓度"=→"COD母液浓度":dbl, "加标体积"=→"COD加标体积":dbl, "加标回收率"=→"COD加标回收率":dbl)
  n221 = Obtain Queue(max queue size (-1, unlimited)=-1 ("队列最大值（-1，无限）"), name (unnamed)="写入" ("名称（未命名）"), element data type=cluster{"starting address":u16, "values":u16[]} {"starting address"=4272, "values"=[]}) -> (queue out=w29:refnum<queue>)  [unwired: 2 in, 2 out]
  n222 = Obtain Queue(name (unnamed)="采配水" ("名称（未命名）"), element data type=cluster{"命令":string, "数据":variant} {"命令"="", "数据"=variant}) -> (queue out=w26:refnum<queue>)  [unwired: 3 in, 2 out]
  n223 = while {
    tunnel: w106 -> [w323]
    tunnel: w62 -> [w322]
    tunnel: w53 -> [w321]
    tunnel: w43 -> [w320]
    tunnel: w33 -> [w319]
    tunnel: w29 -> [w318]
    tunnel: w26 -> [w317]
    tunnel: w16 -> [w316]
    stop <- FALSE stop-if-true
    # "氨氮站号是1，总磷总氮站号是2，COD站号是3"
    n224 = event shown="[15] \"查看\": 值改变" {
      selector: _ -> [_ _ _ _ _ _ _ _ _ _ _ _ _ _ _ _ _]
      dyn-events: _ -> [_ _ _ _ _ _ _ _ _ _ _ _ _ _ _ _ _]
      timeout: _ -> [_ _ _ _ _ _ _ _ _ _ _ _ _ _ _ _ _]
      tunnel: w323 -> [_ _ _ _ _ w347 _ _ _ w423 _ _ _ _ _ _ _]
      tunnel: w322 -> [_ _ _ _ _ _ w361 _ _ w420 _ _ _ _ _ _ _]
      tunnel: w321 -> [_ _ _ _ _ _ _ _ w399 w419 _ _ _ _ _ _ _]
      tunnel: w320 -> [_ _ _ _ _ _ _ _ _ _ _ _ w448 w474 w520 _ _]
      tunnel: w319 -> [_ _ _ _ _ _ _ _ _ _ _ _ _ _ w517 _ _]
      tunnel: w318 -> [_ _ _ _ _ _ _ _ _ _ _ _ _ _ w512 _ _]
      tunnel: w317 -> [_ _ _ _ _ _ _ _ _ _ _ _ _ _ w503 _ _]
      tunnel: w316 -> [_ _ _ _ _ _ _ w379 _ _ _ _ _ _ _ _ _]
      event Timeout {
        n225 = event-data() -> ()  [unwired: 1 in, 3 out]
      }
      event "氨氮量程", "氨氮检出限", "氨氮加标前水样浓度", "氨氮加标水杯定容体积", "氨氮母液浓度", "氨氮加标后水样浓度": Mouse Down {
        n226 = event-data() -> ("CtlRef"=w328:refnum<vi>)  [unwired: 1 in, 7 out]
        n227 = property class="DigNum (严格)"(reference=w328) -> (reference out=w326:refnum<vi>, "Value"=w327:dbl)  [unwired: 1 in, 1 out]
        n228 = call "数字键盘.vi"("OldNumber"=w327) -> ("NewNumber"=w325:sgl)
        n229 = property class="DigNum (严格)"(reference=w326, "Val(Sgnl)"=w325) -> ()  [unwired: 1 in, 2 out]
      }
      event "总磷母液浓度", "总磷加标水杯定容体积", "总磷加标后水样浓度", "总磷加标前水样浓度", "总磷检出限", "总磷量程": Mouse Down {
        n230 = event-data() -> ("CtlRef"=w332:refnum<vi>)  [unwired: 1 in, 7 out]
        n231 = property class="DigNum (严格)"(reference=w332) -> (reference out=w330:refnum<vi>, "Value"=w331:dbl)  [unwired: 1 in, 1 out]
        n232 = call "数字键盘.vi"("OldNumber"=w331) -> ("NewNumber"=w329:sgl)
        n233 = property class="DigNum (严格)"(reference=w330, "Val(Sgnl)"=w329) -> ()  [unwired: 1 in, 2 out]
      }
      event "总氮母液浓度", "总氮加标水杯定容体积", "总氮加标后水样浓度", "总氮加标前水样浓度", "总氮检出限", "总氮量程": Mouse Down {
        n234 = event-data() -> ("CtlRef"=w336:refnum<vi>)  [unwired: 1 in, 7 out]
        n235 = property class="DigNum (严格)"(reference=w336) -> (reference out=w334:refnum<vi>, "Value"=w335:dbl)  [unwired: 1 in, 1 out]
        n236 = call "数字键盘.vi"("OldNumber"=w335) -> ("NewNumber"=w333:sgl)
        n237 = property class="DigNum (严格)"(reference=w334, "Val(Sgnl)"=w333) -> ()  [unwired: 1 in, 2 out]
      }
      event "COD母液浓度", "COD加标水杯定容体积", "COD加标后水样浓度", "COD加标前水样浓度", "COD检出限", "COD量程": Mouse Down {
        n238 = event-data() -> ("CtlRef"=w340:refnum<vi>)  [unwired: 1 in, 7 out]
        n239 = property class="DigNum (严格)"(reference=w340) -> (reference out=w338:refnum<vi>, "Value"=w339:dbl)  [unwired: 1 in, 1 out]
        n240 = call "数字键盘.vi"("OldNumber"=w339) -> ("NewNumber"=w337:sgl)
        n241 = property class="DigNum (严格)"(reference=w338, "Val(Sgnl)"=w337) -> ()  [unwired: 1 in, 2 out]
      }
      event "氨氮量程", "氨氮检出限", "氨氮加标前水样浓度", "氨氮母液浓度", "氨氮加标水杯定容体积", "氨氮加标后水样浓度": Value Change {
        n242 = event-data() -> ()  [unwired: 1 in, 6 out]
        n243 = for {
          tunnel: w347 -> [w359] mode=indexing
          tunnel: [w358] -> w356 mode=indexing
          n244 = property class="DigNum (严格)"(reference=w359) -> ("Value"=w358:dbl)  [unwired: 1 in, 2 out]
        }
        n245 = Index Array(array=w356) -> (element #1=w355:dbl, element #2=w354:dbl, element #3=w341:dbl, element #4=w353:dbl, element #5=w352:dbl, element #6=w350:dbl)  [unwired: 6 in]
        n246 = Bundle By Name(cluster=T8 {"量程"=0.0, "检出限"=0.0, "加标前水样浓度"=0.0, "加标后水样浓度"=0.0, "加标水杯定容体积"=0.0, "加标母液浓度"=0.0, "加标体积"=0.0, "加标回收率"=0.0} ("参数"), "量程"=w355, "检出限"=w354, "加标前水样浓度"=w341, "加标后水样浓度"=w353, "加标水杯定容体积"=w352, "加标母液浓度"=w350) -> (w349:T8)
        n247 = global write "水样浓度全局.vi" "氨氮加标前水样浓度"(w341) -> ()
        n248 = call "加标回收率计算.vi"("参数"=w349) -> ("参数 out"=w348:T8)  [unwired: 10 in]
        n249 = Index Array(array=w347, index #1=6 ("索引")) -> (element #1=w346:refnum<vi>, element #2=w344:refnum<vi>)  [unwired: 1 in]
        n250 = call "质控参数保存.vi"("section"="氨氮质控参数", "参数"=w348) -> ()  [unwired: 9 in, 1 out]
        n251 = Unbundle By Name(w348) -> ("加标体积"=w342:dbl, "加标回收率"=w343:dbl)
        n252 = property class="DigNum (严格)"(reference=w346, "Value"=w342) -> ()  [unwired: 1 in, 2 out]
        n253 = property class="DigNum (严格)"(reference=w344, "Value"=w343) -> ()  [unwired: 1 in, 2 out]
      }
      event "总磷母液浓度", "总磷加标水杯定容体积", "总磷加标后水样浓度", "总磷加标前水样浓度", "总磷检出限", "总磷量程": Value Change {
        n254 = event-data() -> ()  [unwired: 1 in, 6 out]
        n255 = for {
          tunnel: w361 -> [w378] mode=indexing
          tunnel: [w377] -> w375 mode=indexing
          n256 = property class="DigNum (严格)"(reference=w378) -> ("Value"=w377:dbl)  [unwired: 1 in, 2 out]
        }
        n257 = Index Array(array=w375) -> (element #1=w374:dbl, element #2=w373:dbl, element #3=w360:dbl, element #4=w372:dbl, element #5=w371:dbl, element #6=w369:dbl)  [unwired: 6 in]
        n258 = global write "水样浓度全局.vi" "总磷加标前水样浓度"(w360) -> ()
        n259 = Bundle By Name(cluster=T8 {"量程"=0.0, "检出限"=0.0, "加标前水样浓度"=0.0, "加标后水样浓度"=0.0, "加标水杯定容体积"=0.0, "加标母液浓度"=0.0, "加标体积"=0.0, "加标回收率"=0.0} ("参数"), "量程"=w374, "检出限"=w373, "加标前水样浓度"=w360, "加标后水样浓度"=w372, "加标水杯定容体积"=w371, "加标母液浓度"=w369) -> (w368:T8)
        n260 = call "加标回收率计算.vi"("参数"=w368) -> ("参数 out"=w367:T8)  [unwired: 10 in]
        n261 = Index Array(array=w361, index #1=6 ("索引")) -> (element #1=w366:refnum<vi>, element #2=w363:refnum<vi>)  [unwired: 1 in]
        n262 = call "质控参数保存.vi"("section"="总磷质控参数", "参数"=w367) -> ()  [unwired: 9 in, 1 out]
        n263 = Unbundle By Name(w367) -> ("加标体积"=w364:dbl, "加标回收率"=w362:dbl)
        n264 = property class="DigNum (严格)"(reference=w366, "Value"=w364) -> ()  [unwired: 1 in, 2 out]
        n265 = property class="DigNum (严格)"(reference=w363, "Value"=w362) -> ()  [unwired: 1 in, 2 out]
      }
      event "总氮量程", "总氮检出限", "总氮加标前水样浓度", "总氮加标后水样浓度", "总氮加标水杯定容体积", "总氮母液浓度": Value Change {
        n266 = event-data() -> ()  [unwired: 1 in, 6 out]
        n267 = for {
          tunnel: w379 -> [w397] mode=indexing
          tunnel: [w396] -> w394 mode=indexing
          n268 = property class="DigNum (严格)"(reference=w397) -> ("Value"=w396:dbl)  [unwired: 1 in, 2 out]
        }
        n269 = Index Array(array=w394) -> (element #1=w393:dbl, element #2=w392:dbl, element #3=w380:dbl, element #4=w391:dbl, element #5=w390:dbl, element #6=w388:dbl)  [unwired: 6 in]
        n270 = global write "水样浓度全局.vi" "总氮加标前水样浓度"(w380) -> ()
        n271 = Bundle By Name(cluster=T8 {"量程"=0.0, "检出限"=0.0, "加标前水样浓度"=0.0, "加标后水样浓度"=0.0, "加标水杯定容体积"=0.0, "加标母液浓度"=0.0, "加标体积"=0.0, "加标回收率"=0.0} ("参数"), "量程"=w393, "检出限"=w392, "加标前水样浓度"=w380, "加标后水样浓度"=w391, "加标水杯定容体积"=w390, "加标母液浓度"=w388) -> (w387:T8)
        n272 = call "加标回收率计算.vi"("参数"=w387) -> ("参数 out"=w386:T8)  [unwired: 10 in]
        n273 = Index Array(array=w379, index #1=6 ("索引")) -> (element #1=w385:refnum<vi>, element #2=w382:refnum<vi>)  [unwired: 1 in]
        n274 = call "质控参数保存.vi"("section"="总氮质控参数", "参数"=w386) -> ()  [unwired: 9 in, 1 out]
        n275 = Unbundle By Name(w386) -> ("加标体积"=w383:dbl, "加标回收率"=w381:dbl)
        n276 = property class="DigNum (严格)"(reference=w385, "Value"=w383) -> ()  [unwired: 1 in, 2 out]
        n277 = property class="DigNum (严格)"(reference=w382, "Value"=w381) -> ()  [unwired: 1 in, 2 out]
      }
      event "COD母液浓度", "COD加标水杯定容体积", "COD加标后水样浓度", "COD加标前水样浓度", "COD检出限", "COD量程": Value Change {
        n278 = event-data() -> ()  [unwired: 1 in, 6 out]
        n279 = for {
          tunnel: w399 -> [w416] mode=indexing
          tunnel: [w415] -> w413 mode=indexing
          n280 = property class="DigNum (严格)"(reference=w416) -> ("Value"=w415:dbl)  [unwired: 1 in, 2 out]
        }
        n281 = Index Array(array=w413) -> (element #1=w412:dbl, element #2=w411:dbl, element #3=w398:dbl, element #4=w410:dbl, element #5=w409:dbl, element #6=w407:dbl)  [unwired: 6 in]
        n282 = global write "水样浓度全局.vi" "COD加标前水样浓度"(w398) -> ()
        n283 = Bundle By Name(cluster=T8 {"量程"=0.0, "检出限"=0.0, "加标前水样浓度"=0.0, "加标后水样浓度"=0.0, "加标水杯定容体积"=0.0, "加标母液浓度"=0.0, "加标体积"=0.0, "加标回收率"=0.0} ("参数"), "量程"=w412, "检出限"=w411, "加标前水样浓度"=w398, "加标后水样浓度"=w410, "加标水杯定容体积"=w409, "加标母液浓度"=w407) -> (w406:T8)
        n284 = call "加标回收率计算.vi"("参数"=w406) -> ("参数 out"=w405:T8)  [unwired: 10 in]
        n285 = Index Array(array=w399, index #1=6 ("索引")) -> (element #1=w404:refnum<vi>, element #2=w401:refnum<vi>)  [unwired: 1 in]
        n286 = call "质控参数保存.vi"("section"="COD质控参数", "参数"=w405) -> ()  [unwired: 9 in, 1 out]
        n287 = Unbundle By Name(w405) -> ("加标体积"=w402:dbl, "加标回收率"=w400:dbl)
        n288 = property class="DigNum (严格)"(reference=w404, "Value"=w402) -> ()  [unwired: 1 in, 2 out]
        n289 = property class="DigNum (严格)"(reference=w401, "Value"=w400) -> ()  [unwired: 1 in, 2 out]
      }
      event "氨氮调试", "总磷调试", "CODMn调试", "总氮调试": Value Change {
        n290 = event-data() -> ("CtlRef"=w422:refnum<vi>)  [unwired: 1 in, 5 out]
        n291 = property class="Bool"(reference=w422) -> ("Label.Text"=w421:string)  [unwired: 1 in, 2 out]
        n292 = case shown="\"氨氮调试\", 默认" w421 {
          tunnel: w423 -> [w424 _ _ _]
          tunnel: w420 -> [_ w426 w428 _]
          tunnel: w419 -> [_ _ _ w430]
          tunnel: ["氨氮模块" ("标题") "总磷模块" ("标题") "总氮模块" ("标题") "CODMn模块" ("标题")] -> w418
          tunnel: [w424 w426 w428 w430] -> w417
          frame "氨氮调试", Default {
          }
          frame "总磷调试" {
          }
          frame "总氮调试" {
          }
          frame "CODMn调试" {
          }
        }
        n293 = call "加标模块单控对话框.vi"("数组"=w417, "标题"=w418) -> ()  [unwired: 10 in]
      }
      event "氨氮停止", "总磷停止", "CODMn停止", "总氮停止": Value Change {
        n294 = event-data() -> ("CtlRef"=w436:refnum<vi>)  [unwired: 1 in, 5 out]
        n295 = property class="Bool"(reference=w436) -> ("Label.Text"=w435:string)  [unwired: 1 in, 2 out]
        n296 = case shown="\"总氮停止\", \"总磷停止\"" w435 {
          tunnel: [u8 1 ("Slave ID") u8 2 ("Slave ID") u8 3 ("Slave ID")] -> w432
          frame "氨氮停止", Default {
          }
          frame "总氮停止", "总磷停止" {
          }
          frame "CODMn停止" {
          }
        }
        n297 = call "单个写入.vi"("value"=u16 2, "address"=u16 103, "Slave ID"=w432) -> ()  [unwired: 8 in, 1 out]
      }
      event "氨氮排液", "CODMn排液", "总磷排液", "总氮排液": Value Change {
        n298 = event-data() -> ("CtlRef"=w444:refnum<vi>)  [unwired: 1 in, 5 out]
        n299 = property class="Bool"(reference=w444) -> ("Label.Text"=w443:string)  [unwired: 1 in, 2 out]
        n300 = case shown="\"CODMn排液\"" w443 {
          tunnel: [u8 1 ("Slave ID") u8 2 ("Slave ID") u8 3 ("Slave ID")] -> w440
          frame "氨氮排液", Default {
          }
          frame "总氮排液", "总磷排液" {
          }
          frame "CODMn排液" {
          }
        }
        n301 = call "单个写入.vi"("value"=u16 3, "address"=u16 103, "Slave ID"=w440) -> ()  [unwired: 8 in, 1 out]
      }
      event "加标回收": Value Change {
        n302 = event-data() -> ()  [unwired: 1 in, 6 out]
        n303 = flat-sequence {
          tunnel: [w452] -> w451
          tunnel: [w456] -> w450
          tunnel: [w455] -> w449
          tunnel: w448 -> [w453]
          tunnel: w451 -> [w464]
          tunnel: w450 -> [w463]
          tunnel: w449 -> [w462]
          frame #0 {
            n304 = Send Notification(notification=FALSE ("通知"), notifier=w453) -> ()  [unwired: 1 in, 2 out]
            n305 = call "质控启动流程对话框.vi"() -> ("启动模块"=w452:T1, "直接启动"=w455:bool, "常规启动"=w456:bool)  [unwired: 8 in, 1 out]
            "常规启动" <- w456
            "直接启动" <- w455
            "启动模块" <- w452
          }
          frame #1 {
            n306 = Bundle By Name(cluster=T4 {"是否启用仪器"=FALSE, "CODMn"={"启动测量模式"={"测量模式"=enum."水样测量"}, "确定按钮"=FALSE}, "启动模块 3"={"氨氮"=FALSE, "总磷"=FALSE, "总氮"=FALSE, "COD"=FALSE}, "常规启动"=FALSE, "直接启动"=FALSE} ("输出簇"), "是否启用仪器"=TRUE, "启动模块 3"=w464, "常规启动"=w463, "直接启动"=w462) -> (w457:T4)
            "输出簇" <- w457
            n307 = vi-ref "古田户外一体站流程质控自动启动.vi"() -> (w460:refnum<vi>)
            n308 = property class="VI"(reference=w460) -> ("Name"=w461:string, "Exec.State"=w459:T13)  [unwired: 1 in, 2 out]
            n309 = case shown="\"Idle\"" w459 {
              tunnel: w461 -> [_ w472]
              tunnel: w457 -> [_ w471]
              frame "Bad", Default {
              }
              frame "Idle" {
                n310 = Open VI Reference(type specifier VI Refnum (for type only)=refnum<vi> refnum ("类型说明符VI引用句柄（仅用于类型）"), vi path=w472, options=128 ("选项")) -> (vi reference=w473:refnum<vi>, error out=w468:errorcluster)  [unwired: 3 in]
                n311 = call-by-ref "开始异步调用"(reference=w473, error in=w468, "参数"=w471) -> (reference out=w470:refnum<vi>, error out=w469:errorcluster)  [unwired: 11 in]
                n312 = Close Reference(reference=w470, error in (no error)=w469) -> ()  [unwired: 1 out]
              }
            }
          }
        }
      }
      event "平行样测试": Value Change {
        n313 = event-data() -> ()  [unwired: 1 in, 6 out]
        n314 = flat-sequence {
          tunnel: [w479] -> w477
          tunnel: [w481] -> w476
          tunnel: [w480] -> w475
          tunnel: w474 -> [w478]
          tunnel: w477 -> [w488]
          tunnel: w476 -> [w487]
          tunnel: w475 -> [w486]
          frame #0 {
            n315 = Cancel Notification(0:w478) -> ()  [unwired: 1 in, 3 out]
            n316 = call "平行样启动流程对话框.vi"() -> ("启动模块"=w479:cluster{"氨氮1":bool, "总磷1":bool, " COD1":bool}, "直接启动"=w480:bool, "常规启动"=w481:bool)  [unwired: 8 in, 1 out]
            "常规启动 2" <- w481
            "直接启动 2" <- w480
            "启动模块 2" <- w479
          }
          frame #1 {
            n317 = Bundle By Name(cluster=T3 {"是否启用仪器"=FALSE, "CODMn"={"启动测量模式"={"测量模式"=enum."水样测量"}, "确定按钮"=TRUE}, "启动模块"={"氨氮1"=FALSE, "总磷1"=FALSE, " COD1"=FALSE}, "常规启动"=FALSE, "直接启动"=FALSE} ("参数"), "是否启用仪器"=TRUE, "启动模块"=w488, "常规启动"=w487, "直接启动"=w486) -> (w483:T3)
            "输出簇 2" <- w483
            n318 = vi-ref "古田户外一体站流程平行样自动启动.vi"() -> (w484:refnum<vi>)
            n319 = property class="VI"(reference=w484) -> ("Name"=w485:string, "Exec.State"=w482:T13)  [unwired: 1 in, 2 out]
            n320 = case shown="\"Idle\"" w482 {
              tunnel: w485 -> [_ w497]
              tunnel: w483 -> [_ w491]
              frame "Bad", Default {
              }
              frame "Idle" {
                n321 = Open VI Reference(type specifier VI Refnum (for type only)=refnum<vi> refnum ("类型说明符VI引用句柄（仅用于类型）"), vi path=w497, options=128 ("选项")) -> (vi reference=w498:refnum<vi>, error out=w496:errorcluster)  [unwired: 3 in]
                n322 = call-by-ref "开始异步调用"(reference=w498, error in=w496, "参数"=w491) -> (reference out=w493:refnum<vi>, error out=w492:errorcluster)  [unwired: 9 in]
                n323 = Close Reference(reference=w493, error in (no error)=w492) -> ()  [unwired: 1 out]
              }
            }
          }
        }
      }
      event "停止测量": Value Change {
        # "停止采配水、氨氮、总磷总氮、COD、质控"
        n324 = event-data() -> ()  [unwired: 1 in, 6 out]
        n325 = Send Notification(notification=TRUE ("通知"), notifier=w520) -> ()  [unwired: 1 in, 2 out]
        n326 = Enqueue Element(queue=w517, element=cluster{"命令":string, "data":variant} {"命令"="启动", "data"=variant(cluster{"站号":u16, "控制命令输出":u16[]} {"站号"=1, "控制命令输出"=[2816]})} ("元素")) -> ()  [unwired: 2 in, 3 out]
        n327 = call "单个写入.vi"("value"=u16 2, "address"=u16 103, "Slave ID"=u8 1) -> ("error out"=w505:errorcluster)  [unwired: 8 in]
        n328 = call "单个写入.vi"("Error in"=w505, "value"=u16 2, "address"=u16 103, "Slave ID"=u8 2) -> ("error out"=w499:errorcluster)  [unwired: 7 in]
        n329 = Bundle By Name(cluster=cluster{"starting address":u16, "values":u16[]} {"starting address"=0, "values"=[]}, "starting address"=u16 4608, "values"=u16[] [11]) -> (w514:cluster{"starting address":u16, "values":u16[]})
        n330 = Enqueue Element At Opposite End(queue=w503, element=T12 {"命令"="单个写入", {"starting address"=300, "holding register value"=2}} ("元素")) -> ()  [unwired: 2 in, 3 out]
        n331 = call "单个写入.vi"("Error in"=w499, "value"=u16 2, "address"=u16 103, "Slave ID"=u8 3) -> ()  [unwired: 7 in, 1 out]
        n332 = Enqueue Element(queue=w512, element=w514) -> ()  [unwired: 2 in, 3 out]
      }
      event "查看": Value Change {
        n333 = event-data() -> ()  [unwired: 1 in, 6 out]
        n334 = property on="窗格" class="Pane"("Origin"=T6 {"Horizontal"=0, "Vertical"=550} ("原点")) -> ()  [unwired: 2 in, 2 out]
      }
      event "返回": Value Change {
        n335 = event-data() -> ()  [unwired: 1 in, 6 out]
        n336 = property on="窗格" class="Pane"("Origin"=T6 {"Horizontal"=0, "Vertical"=0} ("原点")) -> ()  [unwired: 2 in, 2 out]
      }
    }
  }
  n337 = Build Array("时间" ("table"), "参数" ("table"), "加标前水样测试时间" ("table"), "加标前水样浓度值" ("元素"), "加标后水样浓度值" ("元素"), "加标母液浓度值" ("元素"), "加标体积" ("元素"), "加标水杯定容体积" ("元素"), "加标回收率" ("元素")) -> (→"columns":string[])
  n338 = call-dynamic "Close Session.vi"("error in (no error)"=w50, "MB_Serial session"=w1) -> ()  [unwired: 9 in, 1 out]
